vi "Create Plugin.vi"() -> ()   [LabVIEW 2021, in "Python Orchestration.lvlib"]
uses:
  Python Orchestration.lvlib
panel:
  out "Configuration Valid":bool=TRUE
  out "Logic Valid":bool=TRUE
  out "Logic Entry":string
  out "Configuration Entry":string
  in  "Configuration Parameters":string[](array[string])
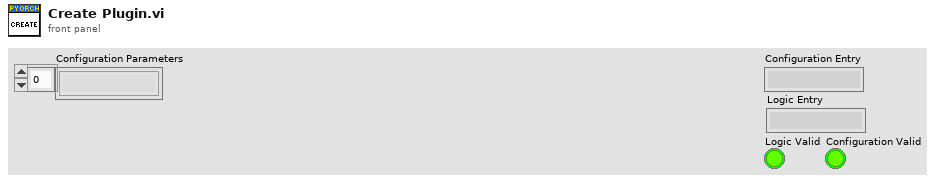
[diagram p1: front panel]
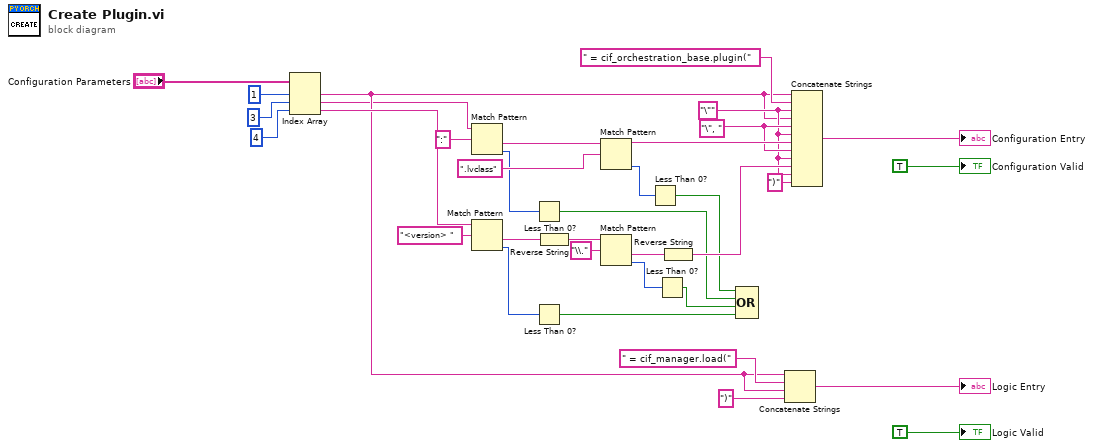
[diagram p0: block diagram]
diagram:
  w23 = "\", "
  w14 = "\""
  n1 = Index Array(array="Configuration Parameters", index #1=1 ("index"), index #2=3 ("index"), index #3=4 ("index")) -> (element #1=w11:string, element #2=w5:string, element #3=w21:string)
  n2 = Match Pattern(string=w5, regular expression=":") -> (after substring=w26:string, offset past match=w9:i32)  [unwired: 1 in, 2 out]
  n3 = Match Pattern(string=w21, regular expression="<version> ") -> (after substring=w19:string, offset past match=w7:i32)  [unwired: 1 in, 2 out]
  n4 = Less Than 0?(x=w9) -> (x < 0?=w2:bool)
  n5 = Less Than 0?(x=w7) -> (x < 0?=w4:bool)
  n6 = Reverse String(1:w19) -> (0:w18:string)
  n7 = Match Pattern(string=w26, regular expression=".lvclass") -> (before substring=w24:string, offset past match=w8:i32)  [unwired: 1 in, 2 out]
  n8 = Match Pattern(string=w18, regular expression="\\.") -> (after substring=w16:string, offset past match=w6:i32)  [unwired: 1 in, 2 out]
  n9 = Less Than 0?(x=w8) -> (x < 0?=w1:bool)
  n10 = Less Than 0?(x=w6) -> (x < 0?=w3:bool)
  n11 = Reverse String(1:w16) -> (0:w15:string)
  n12 = Compound Arithmetic op=OR(w1, w2, w3, w4) -> ()  [unwired: 1 out]
  n13 = Concatenate Strings(w11, " = cif_manager.load(", w11, ")" ("string")) -> (→"Logic Entry":string)
  n14 = Concatenate Strings(w11, " = cif_orchestration_base.plugin(", w14, w11, w23, w14, w24, w23, w14, w15, w14, ")" ("string")) -> (→"Configuration Entry":string)
  "Logic Valid" <- TRUE
  "Configuration Valid" <- TRUE
